vi "Equalize Histogram.vi"(0 "image in":refnum<class "MSC Image.lvclass">, 5 "error in (no error)":errorcluster) -> (14 "image out":refnum<class "MSC Image.lvclass">, 19 "error out":errorcluster)   [LabVIEW 2014, in "MSC Image.lvclass"]
doc: "Spreads the histogram to its borders."
uses:
  MSC Image.lvclass
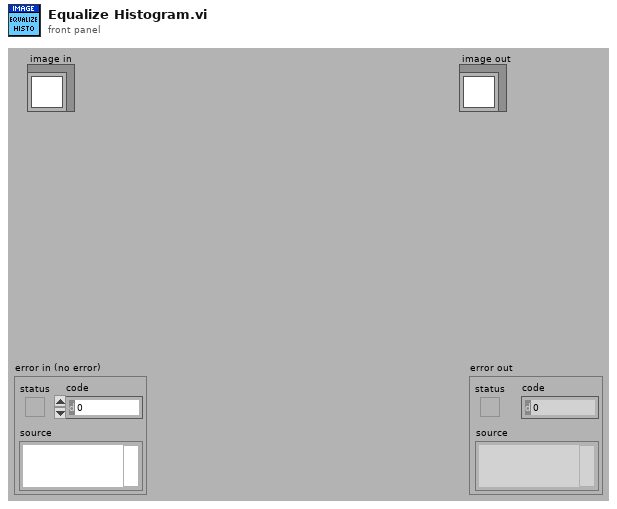
[diagram p1: front panel]
types:
  T1 = typedef "MSC Image.lvclass/Image Type.ctl" = i32
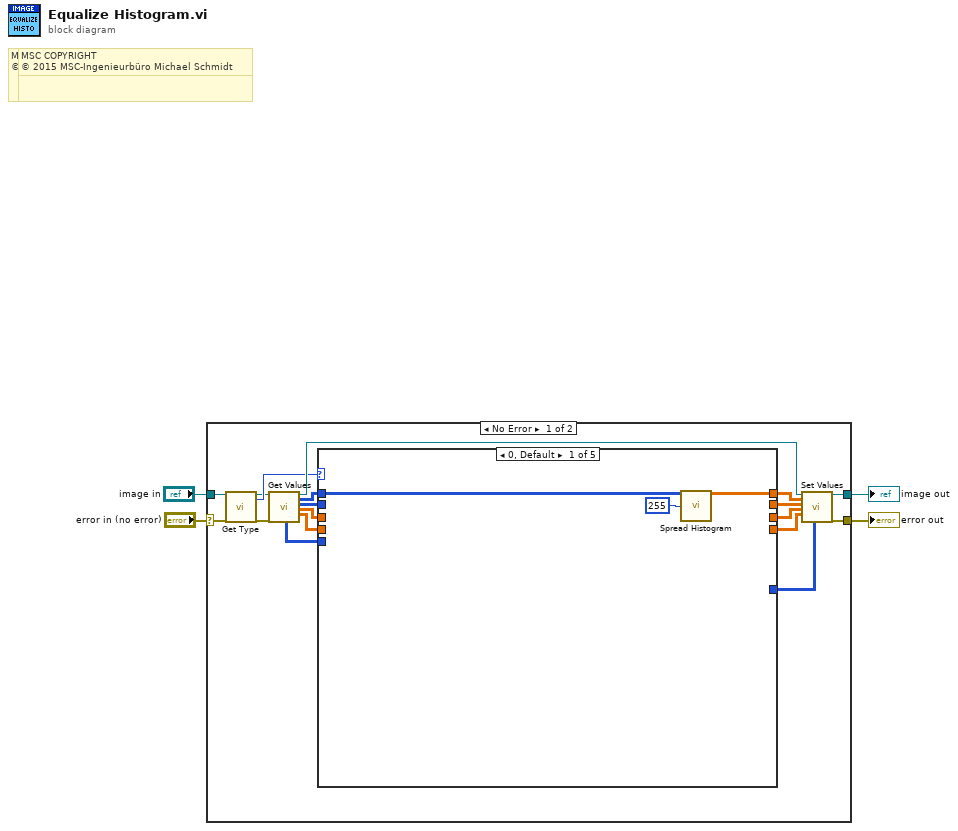
[diagram p0: block diagram]
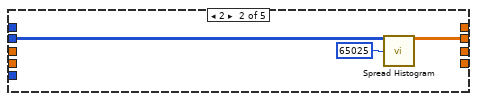
[diagram p2: hidden frame]
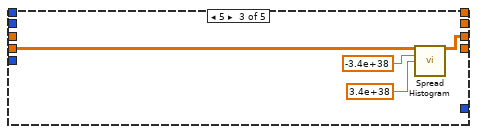
[diagram p3: hidden frame]
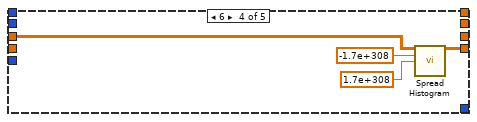
[diagram p4: hidden frame]
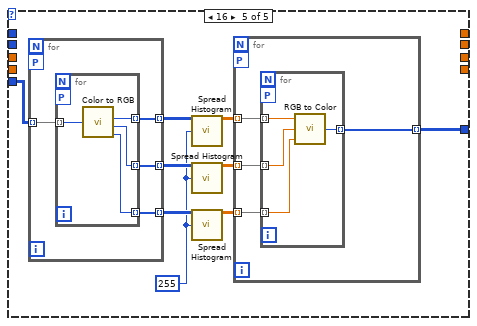
[diagram p5: hidden frame]
diagram:
  # "MSC COPYRIGHT\n© 2016 MSC-Ingenieurbüro Michael Schmidt"
  # "MSC COPYRIGHT\n© 2016 MSC-Ingenieurbüro Michael Schmidt"
  # "MSC COPYRIGHT\n© 2015 MSC-Ingenieurbüro Michael Schmidt"
  # "MSC COPYRIGHT\n© 2015 MSC-Ingenieurbüro Michael Schmidt"
  n1 = case shown="No Error" "error in (no error)" {
    selector: "error in (no error)" -> [w6 w63]
    tunnel: [w20 w63] -> w2
    tunnel: [w21 w62] -> w3
    tunnel: "image in" -> [w8 w62]
    frame No Error {
      n2 = call-dynamic "Get Type.vi"("image in"=w8, "error in (no error)"=w6) -> ("image out"=w7:refnum<class "MSC Image.lvclass">, "Image Type"=w9:T1, "error out"=w5:errorcluster)  [unwired: 15 in]
      n3 = call-dynamic "Get Values.vi"("image in"=w7, "error in (no error)"=w5) -> ("imageData BGR"=w15:u32[][], "image out"=w22:refnum<class "MSC Image.lvclass">, "imageData U8"=w19:u8[][], "imageData U16"=w18:u16[][], "imageData Single"=w17:sgl[][], "imageData Double"=w16:dbl[][])  [unwired: 10 in, 2 out]
      n4 = case shown="0, Default" w9 {
        tunnel: w18 -> [_ w27 _ _ _]
        tunnel: w15 -> [_ _ _ _ w45]
        tunnel: w17 -> [_ _ _ w34 _]
        tunnel: w16 -> [_ _ w30 _ _]
        tunnel: w19 -> [w24 _ _ _ _]
        tunnel: [_ _ _ _ w40] -> w14
        tunnel: [w23 _ _ _ _] -> w13
        tunnel: [_ w26 _ _ _] -> w12
        tunnel: [_ _ w29 _ _] -> w11
        tunnel: [_ _ _ w33 _] -> w10
        frame 0, Default {
          n5 = call "Spread Histogram.vi"("Array in"=w24, "Max"=255) -> ("Array out"=w23:dbl[][])  [unwired: 13 in]
        }
        frame 2 {
          n6 = call "Spread Histogram.vi"("Array in"=w27, "Max"=65025) -> ("Array out"=w26:dbl[][])  [unwired: 13 in]
        }
        frame 5 {
          n7 = call "Spread Histogram.vi"("Array in"=w30, "Min"=-3.4e+38, "Max"=3.4e+38 ("Min")) -> ("Array out"=w29:dbl[][])  [unwired: 12 in]
        }
        frame 6 {
          n8 = call "Spread Histogram.vi"("Array in"=w34, "Min"=-1.7e+308, "Max"=1.7e+308 ("Min")) -> ("Array out"=w33:dbl[][])  [unwired: 12 in]
        }
        frame 16 {
          w41 = 255
          n9 = for {
            tunnel: w45 -> [w57] mode=indexing
            tunnel: [w56] -> w44 mode=indexing
            tunnel: [w55] -> w43 mode=indexing
            tunnel: [w54] -> w42 mode=indexing
            workers-P: _ -> [_]
            n10 = for {
              tunnel: w57 -> [w61] mode=indexing
              tunnel: [w60] -> w56 mode=indexing
              tunnel: [w59] -> w55 mode=indexing
              tunnel: [w58] -> w54 mode=indexing
              workers-P: _ -> [_]
              n11 = call <vilib>:"Color to RGB.vi"("Color"=w61) -> ("R"=w60:u8, "G"=w59:u8, "B"=w58:u8)  [unwired: 1 out]
            }
          }
          n12 = call "Spread Histogram.vi"("Array in"=w44, "Max"=w41) -> ("Array out"=w39:dbl[][])  [unwired: 13 in]
          n13 = call "Spread Histogram.vi"("Array in"=w43, "Max"=w41) -> ("Array out"=w37:dbl[][])  [unwired: 13 in]
          n14 = call "Spread Histogram.vi"("Array in"=w42, "Max"=w41) -> ("Array out"=w38:dbl[][])  [unwired: 13 in]
          n15 = for {
            tunnel: [w49] -> w40 mode=indexing
            tunnel: w39 -> [w48] mode=indexing
            tunnel: w37 -> [w46] mode=indexing
            tunnel: w38 -> [w47] mode=indexing
            workers-P: _ -> [_]
            n16 = for {
              tunnel: [w50] -> w49 mode=indexing
              tunnel: w48 -> [w53] mode=indexing
              tunnel: w46 -> [w52] mode=indexing
              tunnel: w47 -> [w51] mode=indexing
              workers-P: _ -> [_]
              n17 = call <vilib>:"RGB to Color.vi"("B"=w51, "G"=w52, "R"=w53) -> ("Color"=w50:u32)
            }
          }
        }
      }
      n18 = call-dynamic "Set Values.vi"("image in"=w22, "imageData U8"=w13, "imageData U16"=w12, "imageData Single"=w11, "imageData Double"=w10, "imageData BGR"=w14) -> ("image out"=w21:refnum<class "MSC Image.lvclass">, "error out"=w20:errorcluster)  [unwired: 12 in]
    }
    frame Error {
    }
  }
  "error out" <- w2
  "image out" <- w3
